vi "Get User level and name.vi"(11 "UserDetails":string[][](array[string])) -> (3 "UserL&N":string[][](array[string]))   [LabVIEW 2018]
doc: "Get UserLevel and UserName"
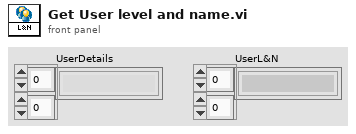
[diagram p1: front panel]
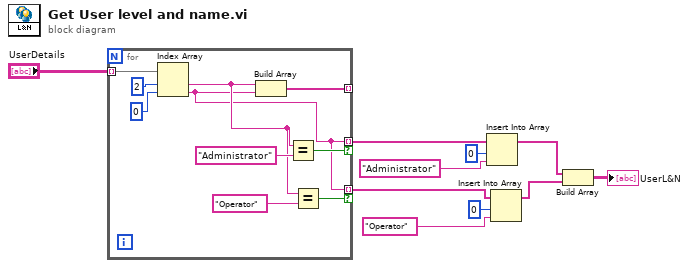
[diagram p0: block diagram]
diagram:
  n1 = for {
    tunnel: "UserDetails" -> [w20] mode=indexing
    tunnel: [w19] -> _ mode=indexing
    tunnel: [w12] -> w9 mode=indexing if=w15
    tunnel: [w12] -> w6 mode=indexing if=w11
    n2 = Index Array(array=w20, index #1=2 ("disabled index (col)"), index #2=0 ("index (col)")) -> (element #1=w13:string, element #2=w12:string)
    n3 = Build Array(w13, w12) -> (w19:string[])
    n4 = Equal?(x=w13, y="Administrator") -> (x = y?=w15:bool)
    n5 = Equal?(x=w13, y="Operator") -> (x = y?=w11:bool)
  }
  n6 = Insert Into Array(array=w9, index=0, new element="Administrator") -> (w3:string[])
  n7 = Insert Into Array(array=w6, index=0, new element="Operator" ("y")) -> (w2:string[])
  n8 = Build Array(w3, w2) -> (→"UserL&N":string[][])
